vi "setImageNumber.vi"(8 "error in (no error)":errorcluster, 9 "Path":path, 10 "imageNumber":i32, 11 "CameraManager in":refnum<class "CameraManager.lvclass">) -> (0 "error out":errorcluster, 3 "CameraManager out":refnum<class "CameraManager.lvclass">)   [LabVIEW 2009, in "iManagement.lvlib" / "CameraManager.lvclass"]
uses:
  CameraManager.lvclass
  CameraManager.lvclass/CameraManager.ctl
  Hal/Channels/Camera/CameraController.lvclass
  Hal/Channels/Camera/CameraEventsManager/CameraEventsManger.lvclass
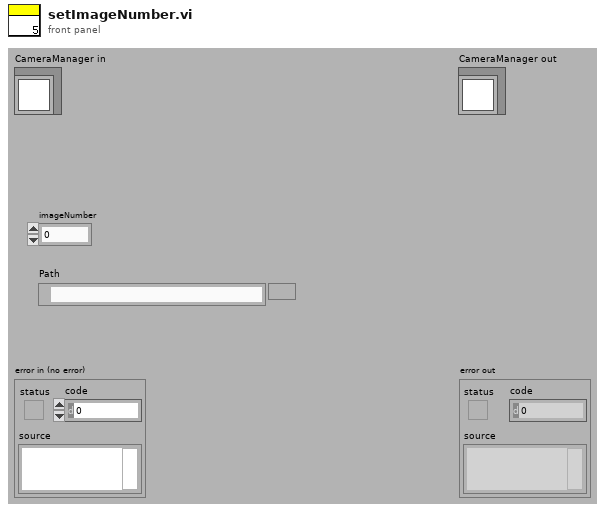
[diagram p1: front panel]
types:
  T1 = cluster{"settingsFrontEndEvents":cluster{"loadSettingsFromPath":refnum<user-event>, "lookUpElementEvent":refnum<user-event>, "saveSettings":refnum<user-event>, "loadSettings":refnum<user-event>, "close":refnum<user-event>, "replaceElement":refnum<user-event>, "findParentNodes":refnum<user-event>, "createNode":refnum<user-event>}, "settingBackEndEvents":cluster{"defaultSettingsPathRequest":refnum<user-event>, "searchResultEvent":refnum<user-event>, "settingsSaved":refnum<user-event>, "settingsLoaded":refnum<user-event>, "foundParentNode":refnum<user-event>}}
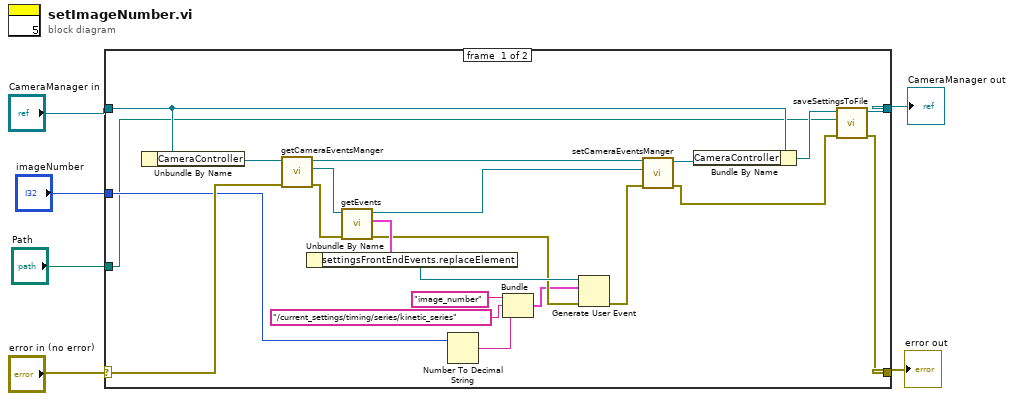
[diagram p0: block diagram]
diagram:
  n1 = case shown="No Error" "error in (no error)" {
    selector: "error in (no error)" -> [w22 w30]
    tunnel: [w7 w30] -> w4
    tunnel: [w10 w29] -> w5
    tunnel: "CameraManager in" -> [w25 w29]
    tunnel: "imageNumber" -> [w13 _]
    tunnel: "Path" -> [w9 _]
    frame #0 {
      n2 = Unbundle By Name(w25) -> ("CameraController"=w26:refnum<class "CameraController.lvclass">)
      n3 = call-dynamic "getCameraEventsManger.vi"("error in (no error)"=w22, "CameraController.lvclass in"=w26) -> ("error out"=w27:errorcluster, "Hardware:Channels.lvlib:CameraEventsManger.lvclass"=w28:refnum<class "CameraEventsManger.lvclass">, "CameraController.lvclass out"=w24:refnum<class "CameraController.lvclass">)  [unwired: 7 in]
      n4 = call-dynamic "getEvents.vi"("error in (no error)"=w27, "CameraEventsManger in"=w28) -> ("error out"=w18:errorcluster, "settingsEvents"=w20:T1, "CameraEventsManger out"=w21:refnum<class "CameraEventsManger.lvclass">)  [unwired: 5 in, 2 out]
      n5 = Unbundle By Name(w20) -> ("settingsFrontEndEvents.replaceElement"=w19:refnum<user-event>)
      n6 = Number To Decimal String(number=w13) -> (decimal integer string=w14:string)  [unwired: 1 in]
      n7 = Bundle("image_number", "/current_settings/timing/series/kinetic_series", w14) -> (w12:cluster{string, string, string})  [unwired: 1 in]
      n8 = Generate User Event(user event=w19, event data cluster=w12, error in=w18) -> (error out=w17:errorcluster)  [unwired: 1 out]
      n9 = call-dynamic "setCameraEventsManger.vi"("error in (no error)"=w17, "Hardware:Channels.lvlib:CameraEventsManger.lvclass"=w21, "CameraController.lvclass in"=w24) -> ("error out"=w8:errorcluster, "CameraController.lvclass out"=w23:refnum<class "CameraController.lvclass">)  [unwired: 7 in]
      n10 = Bundle By Name(cluster=w25, "CameraController"=w23) -> (w11:refnum<class "CameraManager.lvclass">)
      n11 = call "saveSettingsToFile.vi"("error in (no error)"=w8, "Path"=w9, "CameraManager in"=w11) -> ("error out"=w7:errorcluster, "CameraManager out"=w10:refnum<class "CameraManager.lvclass">)  [unwired: 7 in]
    }
    frame #1 {
    }
  }
  "error out" <- w4
  "CameraManager out" <- w5
